vi "N-Double FFT Mesurament (N-Parametric) Test.vi"() -> ()   [LabVIEW 2014]
uses:
  <vilib>/Platform/TimedLoop/XDataNode/timing_clust.ctl
  <vilib>/Platform/TimedLoop/XDataNode/nitl_modes.ctl
  <vilib>/Platform/TimedLoop/XDataNode/wakeup.ctl
  <vilib>/rvi/Analysis/measure/FFT/simModelSupport/niFPGA FFT Streaming Sim Properties.ctl
  <vilib>/rvi/Analysis/measure/FFT/simModelSupport/niFPGA FFT Sim Stream Group Properties.ctl
  <vilib>/rvi/Analysis/measure/FFT/simModelSupport/niFPGA FFT Sim Types.ctl
  <vilib>/rvi/Analysis/measure/FFT/simModelSupport/niFpgaFFTSimArithmeticProperties.ctl
  <vilib>/rvi/Analysis/measure/FFT/simModelSupport/niFpgaFFTSimDfxp.ctl
  <vilib>/fxp/LVFixedPointQuantizationPolicyTypeDef.ctl
  <vilib>/rvi/Analysis/measure/FFT/XNode/niFpgaFFTButterflyDelays.ctl
  <vilib>/rvi/Emulation/niFpgaSctlEmulationGetInTimedLoop.vi
  <vilib>/rvi/Emulation/niFpgaEmulationReportErrorSimple.vi
  <vilib>/rvi/Emulation/niFpgaGetClockAttributes.vi
  <vilib>/rvi/Emulation/niFpgaCriticalErrorInLSC.vi
  <vilib>/rvi/Emulation/niFpgaEmulationIsFPGAContextNoSignature.vi
  <vilib>/rvi/DataTransferAndStorage/Container/Common/niFpgaContainerGetUniqueNameForEmu.vi
  <vilib>/rvi/Memory/Memory_Emulation/niFpgaMemoryEmulationCacheClearOnFirstRun.vi
  <vilib>/rvi/Memory/Memory_Emulation/nirvimemoryEmulationManagerCache_MakeExclusive.vi
  <vilib>/rvi/Memory/Memory_Emulation/niFpgaMemoryEmulationValidateCache.vi
  <vilib>/rvi/Memory/Memory_Emulation/nirvimemoryEmulationManagerCache_InsertValue.vi
  <vilib>/Utility/error.llb/Clear Errors.vi
  <vilib>/rvi/Memory/Memory_Emulation/nirvimemoryEmulationManagerCache_ReleaseExclusive.vi
  <vilib>/rvi/Memory/Memory_Emulation/nirvimemoryEmulationManagerCache_GetValue.vi
  <vilib>/rvi/Memory/Memory_Emulation/nirvimemoryEmulationManagerCache_SetValue.vi
  <vilib>/rvi/Emulation/niFpgaProcessEmulError.vi
  <vilib>/rvi/errors/niFpgaSetErrorForExecOnDevCompSimple.vi
  <vilib>/rvi/eio/common/nirviEmuReportErrorAndStop.vi
  <vilib>/rvi/FIFO/Fifo_Resource/nirvififoEmulationSetSize.vi
  <vilib>/rvi/FIFO/Fifo_Resource/nirviFifoEmulationQueueMgr.vi
  <instcachedir>/0/nirviFifoEmulationQueueMgr_E5CAEC123FF24DC58D834DCA3CDAA9B5.lvgen/nirviFifoEmulationQueueMgr_E5CAEC123FF24DC58D834DCA3CDAA9B5_010.vi
  <vilib>/rvi/FIFO/Fifo_Resource/nirvififoEmulationCreateLock.vi
  <vilib>/rvi/FIFO/Fifo_Resource/nirvififoEmulationObtainLock.vi
  <vilib>/rvi/FIFO/Fifo_Resource/nirvififoEmulationReleaseLock.vi
  <vilib>/rvi/occurrence/nirviWaitOnOccurrenceBase.vi
  <vilib>/rvi/errors/nirviReportUnexpectedCaseInternalError.vi
  <vilib>/rvi/errors/nirviReportUnexpectedCaseInternalError (U32).vi
  <vilib>/rvi/FIFO/Fifo_Resource/nirvififoEmulationDetermineInputValidOut.vi
  <vilib>/rvi/Memory/Memory_Emulation/nirvimemoryFastEmulation.vi
  <vilib>/rvi/Memory/Memory_Emulation/nirvimemoryEmulation.vi
  <vilib>/rvi/eio/common/nirviEmuTemplateMethod_errors.vi
  <vilib>/rvi/Analysis/measure/FFT/simModelSupport/niFpgaFFTSimModelStreamingCore.vi
  <vilib>/rvi/interface/RandomDataEmulation/niFpgaRandomDataHandleErrors.vi
  <vilib>/Platform/TimedLoop/XDataNode/XDataNode.xnode
  <vilib>/rvi/DataTransferAndStorage/Container/XNode/niFpgaContainer.xnode
  <vilib>/rvi/DataTransferAndStorage/Register/Emulation/niFpgaRegisterEmulation.vi
  <vilib>/rvi/FIFO/Fifo_Resource/nirvififoEmulationRead.vi
  <vilib>/rvi/FIFO/Fifo_Resource/nirvififoEmulationWrite.vi
  <vilib>/eio/EIOMethodNode/EIOMethodNode.xnode
  <vilib>/rvi/Analysis/measure/FFT/XNode/niFpgaFFT.xnode
  <vilib>/rvi/interface/RandomDataEmulation/nirviRandomDataFpgaReadWriteTemplate.vi
  <vilib>/Platform/TimedLoop/XDataNode/XDNodeRunTimeDep.lvlib
panel:
  in  "n":u32=1
  in  "Latency points":u32
  in  "snapshot":bool
  in  "lower limit 2":u32=682
  in  "lower limit 1":u32=57
  in  "upper limit 2":u32=1193
  in  "upper limit 1":u32=568
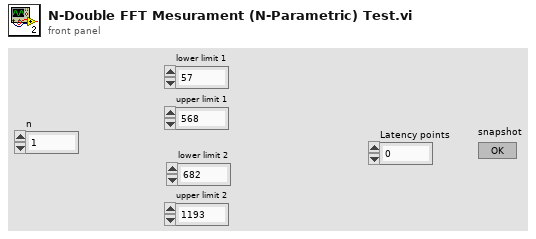
[diagram p1: front panel]
types:
  T1 = typedef "XDNodeRunTimeDep.lvlib/timing_clust.ctl" = cluster{"Expected End [f-1]":u64, "Actual End [f-1]":u64, "Finished Late? [f-1]":bool, "Expected End [i-1]":u64, "Actual End [i-1]":u64, "Finished Late? [i-1]":bool, "Expected Start [i]":u64, "Actual Start [i]":u64, "Expected Start [f]":u64, "Actual Start [f]":u64, "Source Name":string, "Structure Name":string, "Period":i64, "Deadline":i64, "Offset":i64, "Start":i64, "Priority":i32, "Timeout":i32, "Mode":T2, "Wakeup Reason":T3, "Error":errorcluster, "Source Type":string, "Secondary Source Type":string, "Global End Time":u64, "Global Start Time":u64, "Frame Duration":u64, "Iteration Duration":u64, "Assigned CPU":i32, "I/O Scan Engine Mode":u32}
  T2 = typedef "XDNodeRunTimeDep.lvlib/nitl_modes.ctl" = enum32{"No Change", "Process missed periods, maintain original phase", "Discard missed periods, maintain original phase", "Process missed periods, ignore original phase", "Discard missed periods, ignore original phase"}
  T3 = typedef "XDNodeRunTimeDep.lvlib/wakeup.ctl" = enum32{"Normal", "Aborted", "Asynchronous wakeup", "Timing source error", "Timed loop error", "Timeout"}
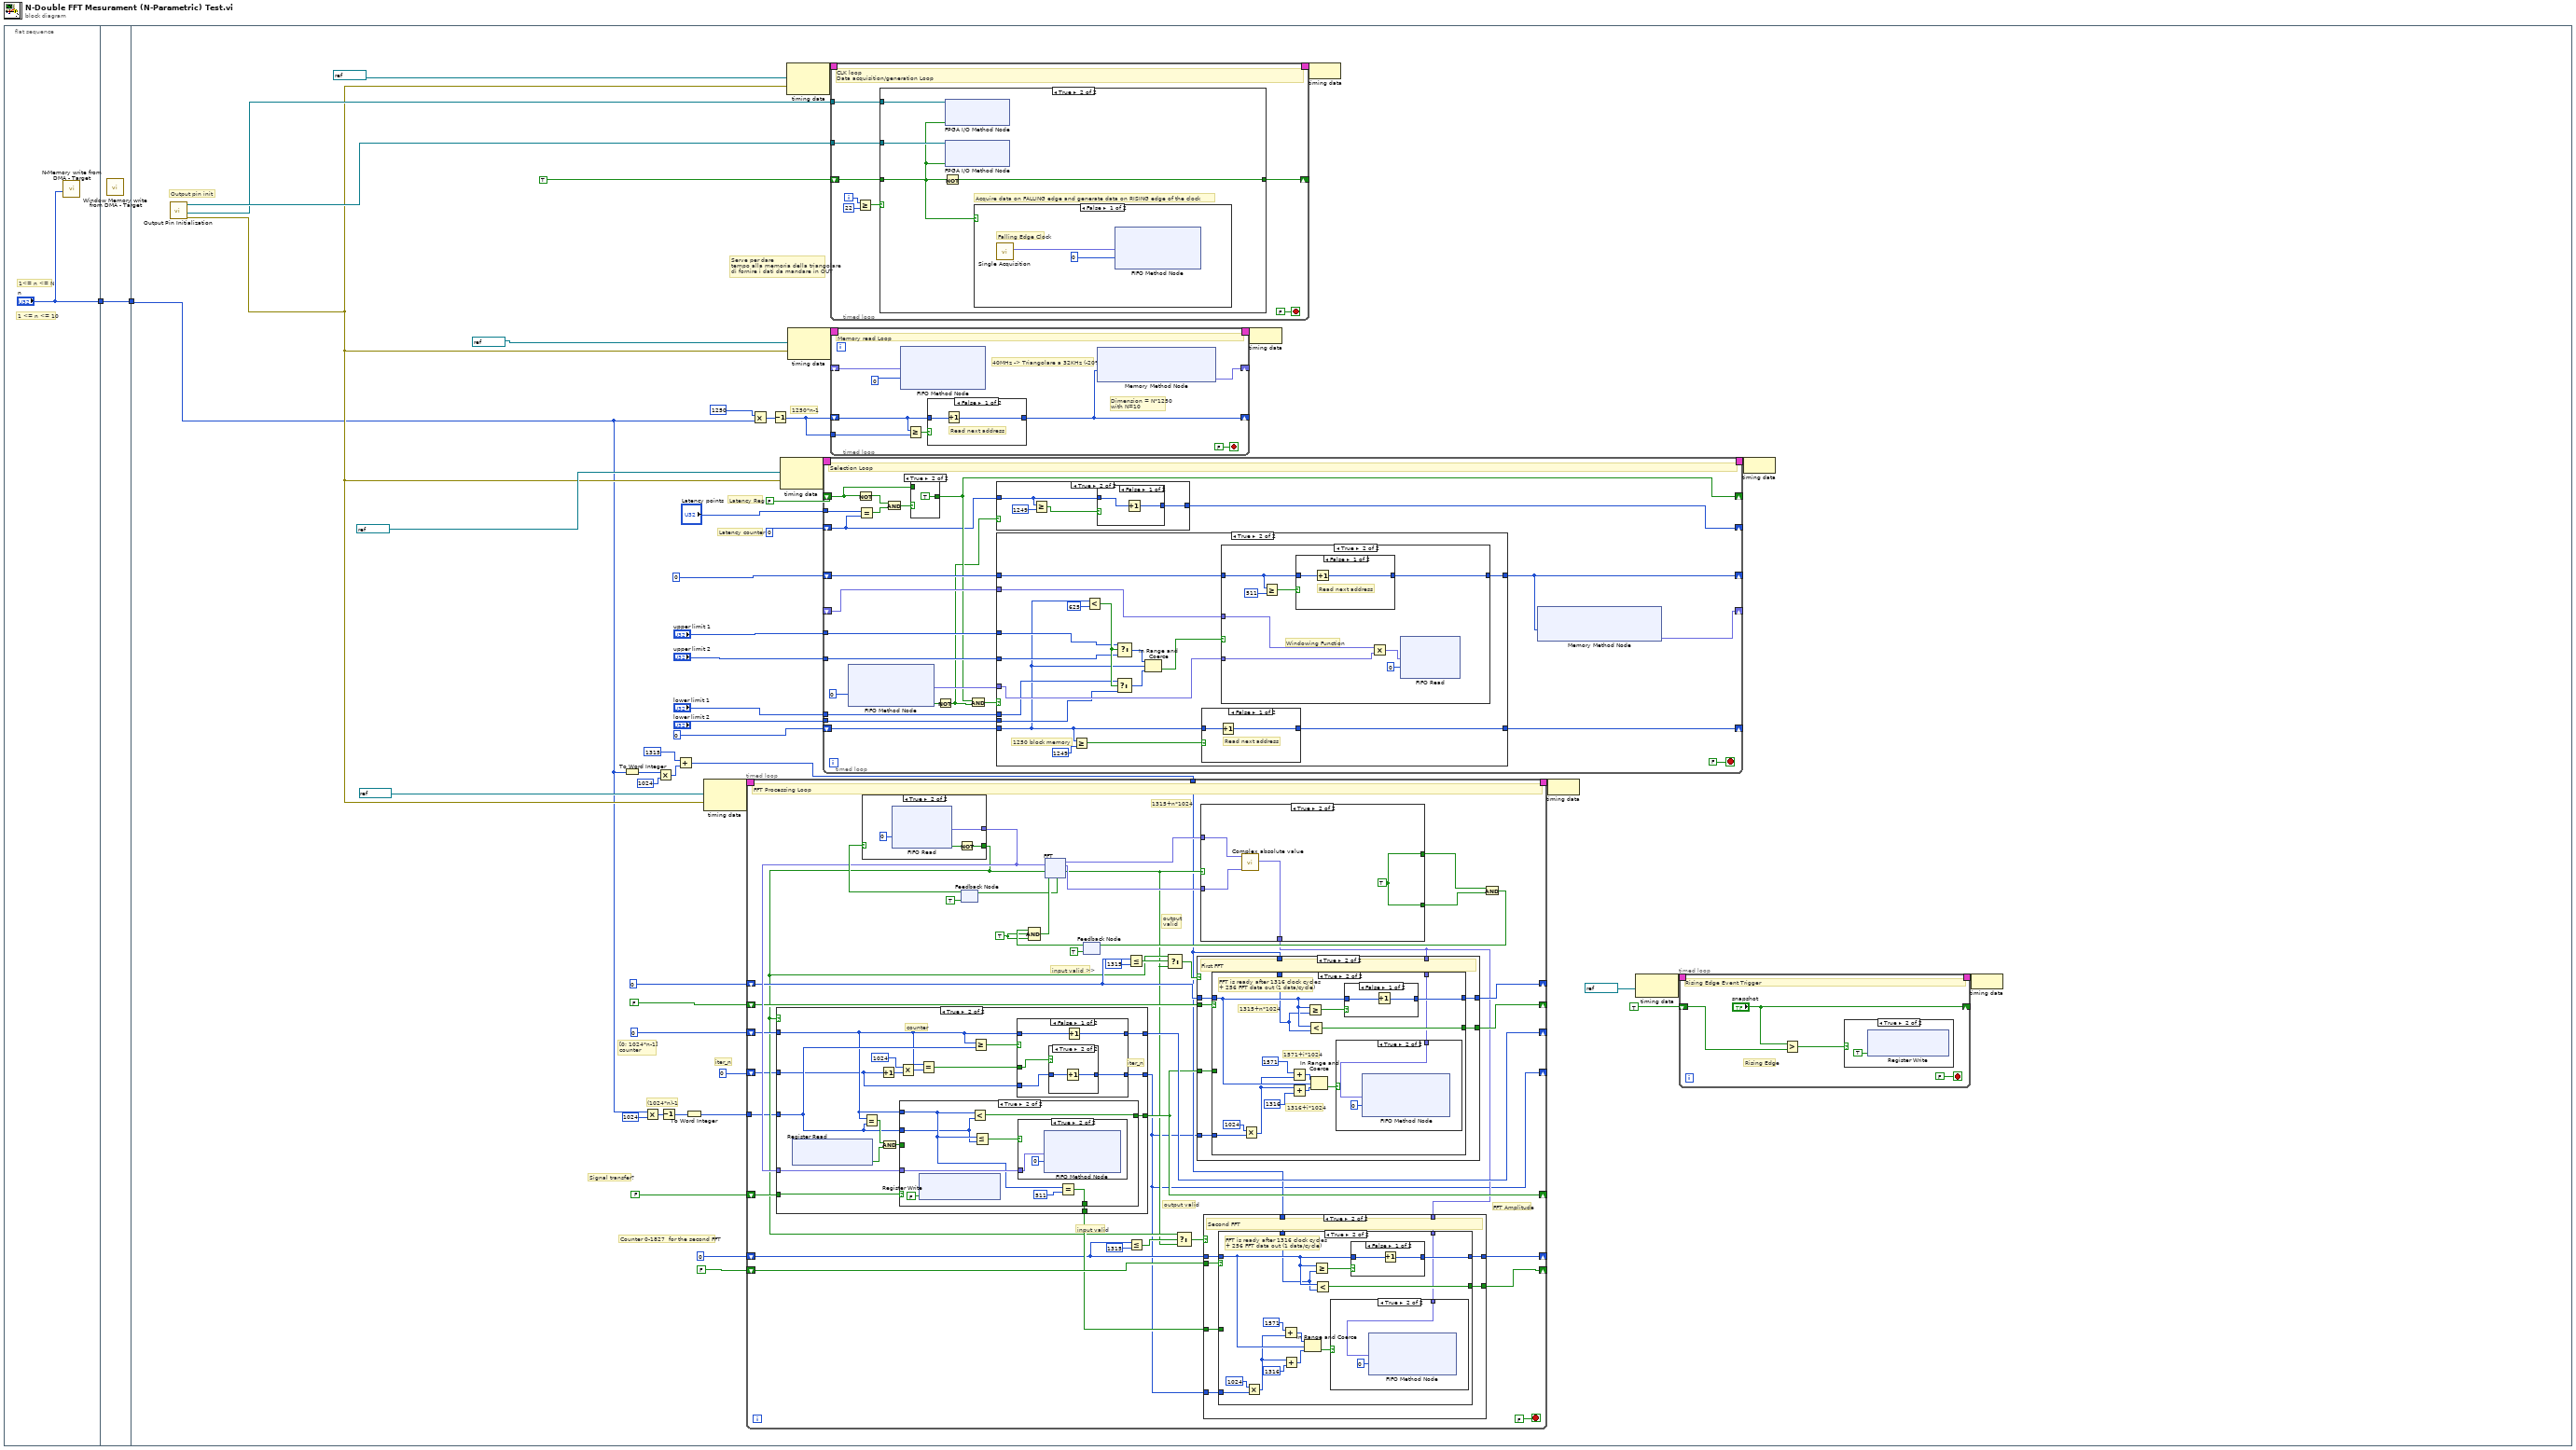
[diagram p0: block diagram]
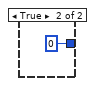
[diagram p4: hidden frame]
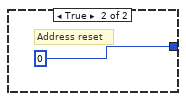
[diagram p8: hidden frame]
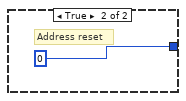
[diagram p9: hidden frame]
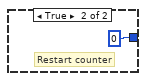
[diagram p13: hidden frame]
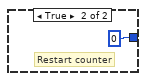
[diagram p17: hidden frame]
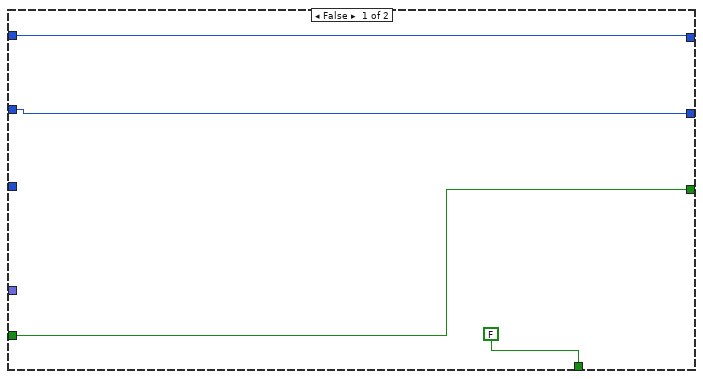
[diagram p18: hidden frame]
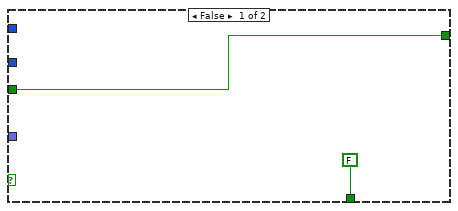
[diagram p19: hidden frame]
diagram:
  n1 = flat-sequence {
    tunnel: ["n"] -> w1
    tunnel: [w4] -> w2
    tunnel: w1 -> [w4]
    tunnel: w2 -> [w6]
    frame #0 {
      # "1 <= n <= 10"
      # "1<= n <= N"
      n2 = call "N-Memory write from DMA - Target.vi"("n"="n") -> ()  [unwired: 11 in]
    }
    frame #1 {
      n3 = call "Window Memory write from DMA - Target.vi"() -> ()  [unwired: 12 in]
    }
    frame #2 {
      # "iter_n"
      # "(1024*n)-1"
      # "1250*n-1"
      # "Serve per dare\ntempo alla memoria della triangolare\ndi fornire i dati da mandare in OUT"
      # "Latency counter"
      # "Latency Reg"
      # "Counter 0-1827  for the second FFT"
      # "[0; 1024*n-1]\ncounter"
      # "Signal transfer?"
      # "Output pin init"
      n4 = call "Output Pin Initialization.vi"() -> ("error out"=w37:errorcluster, "I/O Out Clock DAC (pin16)"=w41:refnum<k21>, "I/O Out Clock ADC (pin17)"=w42:refnum<k21>)  [unwired: 8 in]
      n5 = To Word Integer(number=w6) -> (16bit integer=w7:i16)
      n6 = Multiply(x=w6, y=u32 1024) -> (x*y=w14:u32)
      n7 = Multiply(x=w7, y=i16 1024) -> (x*y=w9:i16)
      n8 = Decrement(x=w14) -> (x-1=w13:u32)
      n9 = Add(x=i16 1315 ("y"), y=w9) -> (x+y=w5:i16)
      n10 = To Word Integer(number=w13) -> (16bit integer=w12:i16)
      n11 = node-c288(refnum<k21> "40MHz" ("Source Name"), w37) -> (w49:T1)
      n12 = timed-loop {
        timing: w49 -> [_]
        timing-out: [_] -> w48
        shift-right: [w163] -> _
        shift-left: FALSE -> [w166]
        shift-right: [w167] -> _
        shift-left: i16 0 -> [w164]
        shift-right: [w162] -> _
        shift-left: FALSE -> [w161]
        shift-right: [w160] -> _
        shift-left: i16 0 -> [w158]
        shift-right: [w155] -> _
        shift-left: i16 0 -> [w148]
        shift-right: [w152] -> _
        shift-left: FALSE -> [w153]
        tunnel: w12 -> [w143]
        shift-right: [w140] -> _
        shift-left: i16 0 -> [w142]
        tunnel: w5 -> [w141]
        stop <- FALSE stop-if-true
        w144 = TRUE
        # "1315+n*1024"
        # "output valid"
        # "input valid"
        # "FFT Amplitude"
        # "output\nvalid"
        # "input valid >>"
        # "FFT Processing Loop"
        n13 = feedback #1(TRUE ("ready for input")) -> (w179:bool)
        n14 = case shown="True" w179 {
          tunnel: [FALSE w320] -> w147
          tunnel: [fxp<+/-,12,12> 0.0 ("Element") w317] -> w165
          frame False {
            # "RMS is not ready for new input"
          }
          frame True {
            n15 = xnode ("FIFO Read")("Timeout"=0) -> ("Element"=w317:fxp<+/-,12,12>, "Timed Out?"=w319:bool)  [unwired: 1 in, 1 out]
            n16 = Not(x=w319) -> (.not. x?=w320:bool)
          }
        }
        n17 = case shown="True" w147 {
          tunnel: w164 -> [w245 w249]
          tunnel: [w245 w261] -> w167
          tunnel: w166 -> [w244 w257]
          tunnel: [w244 w258] -> w163
          tunnel: w165 -> [_ w256]
          tunnel: [FALSE w254] -> w151
          tunnel: w143 -> [_ w253]
          tunnel: w142 -> [w242 w247]
          tunnel: [w242 w246] -> w140
          frame False {
          }
          frame True {
            # "iter_n"
            # "counter"
            n18 = xnode ("Register Read")() -> ("Data"=w255:bool)  [unwired: 1 in, 1 out]
            n19 = Equal?(x=w249, y=w253) -> (x = y?=w260:bool)
            n20 = Increment(x=w247) -> (x+1=w252:i16)
            n21 = And(x=w260, y=w255) -> (x .and. y?=w259:bool)
            n22 = Multiply(x=i16 1024, y=w252) -> (x*y=w250:i16)
            n23 = case shown="True" w257 {
              tunnel: w259 -> [w264 _]
              tunnel: w249 -> [_ w266]
              tunnel: [w264 w272] -> w258
              tunnel: w256 -> [_ w267]
              tunnel: [FALSE w268] -> w254
              tunnel: w253 -> [_ w265]
              frame False {
              }
              frame True {
                n24 = xnode ("Register Write")("Data"=FALSE) -> ()  [unwired: 1 in, 1 out]
                n25 = Less?(x=w266, y=w265) -> (x < y?=w272:bool)
                n26 = Less Or Equal?(x=w266, y=w265) -> (x <= y?=w271:bool)
                n27 = case shown="True" w271 {
                  tunnel: w267 -> [_ w273]
                  frame False {
                  }
                  frame True {
                    n28 = xnode ("FIFO Method Node")("Element"=w273, "Timeout"=0) -> ()  [unwired: 1 in, 2 out]
                  }
                }
                n29 = Equal?(x=w266, y=i16 511) -> (x = y?=w268:bool)
              }
            }
            n30 = Equal?(x=w249, y=w250) -> (x = y?=w248:bool)
            n31 = Greater Or Equal?(x=w249, y=w253) -> (x >= y?=w262:bool)
            n32 = case shown="False" w262 {
              tunnel: w249 -> [w279 _]
              tunnel: [w278 w283] -> w261
              tunnel: w248 -> [w276 _]
              tunnel: w247 -> [w277 _]
              tunnel: [w275 w283] -> w246
              frame False {
                n33 = case shown="True" w276 {
                  tunnel: w277 -> [w280 w282]
                  tunnel: [w280 w281] -> w275
                  frame False {
                  }
                  frame True {
                    n34 = Increment(x=w282) -> (x+1=w281:i16)
                  }
                }
                n35 = Increment(x=w279) -> (x+1=w278:i16)
              }
              frame True {
                w283 = i16 0
                # "Restart counter"
              }
            }
          }
        }
        n36 = feedback #2(TRUE) -> (w175:bool)
        n37 = Compound Arithmetic op=AND(w175, w144, w144) -> (w174:bool)
        n38 = xnode "FFT"("real data in"=w165, "input valid"=w147, "ready for output"=w174) -> ("ready for input"=w173:bool, "real data out"=w172:fxp<+/-,22,22>, "imaginary data out"=w171:fxp<+/-,22,22>, "output valid"=w145:bool)  [unwired: 2 in, 1 out]
        n39 = feedback-in #1(w173) -> ()
        n40 = Less Or Equal?(x=w158, y=i16 1315) -> (x <= y?=w159:bool)
        n41 = Less Or Equal?(x=w148, y=i16 1315) -> (x <= y?=w149:bool)
        n42 = Select(t=w147, s=w159, f=w145) -> (s? t:f=w156:bool)
        n43 = Select(t=w147, s=w149, f=w145) -> (s? t:f=w146:bool)
        n44 = case shown="True" w145 {
          tunnel: w172 -> [_ w314]
          tunnel: w171 -> [_ w313]
          tunnel: [w310 w311] -> w170
          tunnel: [w310 w311] -> w169
          tunnel: [_ w312] -> w154
          frame False {
            w310 = TRUE
          }
          frame True {
            w311 = TRUE
            n45 = call "Complex absolute value.vi"("Im"=w313, "Re"=w314) -> ("Square Absolute Value"=w312:fxp<+,44,44>)  [unwired: 9 in]
          }
        }
        n46 = case shown="True" w156 {
          tunnel: w163 -> [_ w220]
          tunnel: [w211 w219] -> w162
          tunnel: w161 -> [w211 w218]
          tunnel: w158 -> [w212 w217]
          tunnel: [w212 w216] -> w160
          tunnel: w154 -> [_ w215]
          tunnel: w141 -> [_ w214]
          tunnel: w140 -> [_ w213]
          frame False {
          }
          frame True {
            # "First FFT"
            n47 = case shown="True" w218 {
              tunnel: w220 -> [w222 _]
              tunnel: [w222 w236] -> w219
              tunnel: w217 -> [w221 w231]
              tunnel: [w221 w234] -> w216
              tunnel: w215 -> [_ w232]
              tunnel: w214 -> [_ w230]
              tunnel: w213 -> [_ w224]
              frame False {
              }
              frame True {
                # "1571+i*1024"
                # "1316+i*1024"
                # "1315+n*1024"
                # "FFT is ready after 1316 clock cycles\n+ 256 FFT data out (1 data/cycle)"
                n48 = Multiply(x=i16 1024 ("upper limit"), y=w224) -> (x*y=w223:i16)
                n49 = Add(x=i16 1571 ("upper limit"), y=w223) -> (x+y=w227:i16)
                n50 = Add(x=w223, y=i16 1316) -> (x+y=w229:i16)
                n51 = Greater Or Equal?(x=w231, y=w230) -> (x >= y?=w235:bool)
                n52 = Less?(x=w231, y=w230) -> (x < y?=w236:bool)
                n53 = In Range and Coerce(upper limit=w227, x=w231, lower limit=w229) -> (In Range?=w233:bool)  [unwired: 1 out]
                n54 = case shown="True" w233 {
                  tunnel: w232 -> [_ w238]
                  frame False {
                  }
                  frame True {
                    n55 = xnode ("FIFO Method Node")("Element"=w238, "Timeout"=0) -> ()  [unwired: 1 in, 2 out]
                  }
                }
                n56 = case shown="False" w235 {
                  tunnel: w231 -> [w240 _]
                  tunnel: [w239 i16 0] -> w234
                  frame False {
                    n57 = Increment(x=w240) -> (x+1=w239:i16)
                  }
                  frame True {
                    # "Restart counter"
                  }
                }
              }
            }
          }
        }
        n58 = case shown="True" w146 {
          tunnel: w151 -> [_ w189]
          tunnel: [w180 w188] -> w152
          tunnel: w153 -> [w180 w187]
          tunnel: w148 -> [w181 w186]
          tunnel: [w181 w185] -> w155
          tunnel: w154 -> [_ w184]
          tunnel: w141 -> [_ w183]
          tunnel: w140 -> [_ w182]
          frame False {
          }
          frame True {
            # "Second FFT"
            n59 = case shown="True" w187 {
              tunnel: w189 -> [w191 _]
              tunnel: [w191 w205] -> w188
              tunnel: w186 -> [w190 w202]
              tunnel: [w190 w203] -> w185
              tunnel: w184 -> [_ w200]
              tunnel: w183 -> [_ w199]
              tunnel: w182 -> [_ w197]
              frame False {
              }
              frame True {
                # "FFT is ready after 1316 clock cycles\n+ 256 FFT data out (1 data/cycle)"
                n60 = Multiply(x=i16 1024 ("upper limit"), y=w197) -> (x*y=w192:i16)
                n61 = Add(x=i16 1571 ("upper limit"), y=w192) -> (x+y=w193:i16)
                n62 = Add(x=w192, y=i16 1316) -> (x+y=w195:i16)
                n63 = In Range and Coerce(upper limit=w193, x=w202, lower limit=w195) -> (In Range?=w201:bool)  [unwired: 1 out]
                n64 = Greater Or Equal?(x=w202, y=w199) -> (x >= y?=w204:bool)
                n65 = Less?(x=w202, y=w199) -> (x < y?=w205:bool)
                n66 = case shown="True" w201 {
                  tunnel: w200 -> [_ w207]
                  frame False {
                  }
                  frame True {
                    n67 = xnode ("FIFO Method Node")("Element"=w207, "Timeout"=0) -> ()  [unwired: 1 in, 2 out]
                  }
                }
                n68 = case shown="False" w204 {
                  tunnel: w202 -> [w209 _]
                  tunnel: [w208 i16 0] -> w203
                  frame False {
                    n69 = Increment(x=w209) -> (x+1=w208:i16)
                  }
                  frame True {
                    # "Restart counter"
                  }
                }
              }
            }
          }
        }
        n70 = Compound Arithmetic op=AND(w170, w169) -> (w168:bool)
        n71 = feedback-in #2(w168) -> ()
      }
      n72 = Multiply(x=u32 1250, y=w6) -> (x*y=w17:u32)
      n73 = Decrement(x=w17) -> (x-1=w16:u32)
      n74 = node-c288(refnum<k21> "40MHz" ("Source Name"), w37) -> (w47:T1)
      n75 = node-c288(refnum<k21> "80MHz" ("Source Name"), w37) -> (w53:T1)
      n76 = node-c288(refnum<k21> "40MHz" ("Source Name"), w37) -> (w51:T1)
      n77 = timed-loop {
        timing: w47 -> [_]
        timing-out: [_] -> w46
        shift-right: [w87] -> _
        shift-left: u32 0 -> [w74]
        tunnel: "upper limit 1" -> [w83]
        tunnel: "upper limit 2" -> [w82]
        tunnel: "lower limit 1" -> [w81]
        tunnel: "lower limit 2" -> [w80]
        shift-right: [w76] -> _
        shift-left: u32 0 -> [w79]
        shift-right: [w77] -> _
        shift-left: _ -> [w78]
        shift-right: [w68] -> _
        shift-left: FALSE -> [w69]
        tunnel: "Latency points" -> [w73]
        shift-right: [w66] -> _
        shift-left: u32 0 -> [w65]
        stop <- FALSE stop-if-true
        # "Selection Loop"
        n78 = xnode ("FIFO Method Node")("Timeout"=0) -> ("Element"=w85:fxp<+/-,12,12>, "Timed Out?"=w86:bool)  [unwired: 1 in, 1 out]
        n79 = Not(x=w69) -> (.not. x?=w72:bool)
        n80 = Equal?(x=w73, y=w65) -> (x = y?=w71:bool)
        n81 = And(x=w72, y=w71) -> (x .and. y?=w70:bool)
        n82 = case shown="True" w70 {
          tunnel: [w97 TRUE] -> w68
          tunnel: w69 -> [w97 _]
          frame False {
          }
          frame True {
          }
        }
        n83 = Not(x=w86) -> (.not. x?=w67:bool)
        n84 = And(x=w68, y=w67) -> (x .and. y?=w75:bool)
        n85 = case shown="True" w67 {
          tunnel: w65 -> [w89 w92]
          tunnel: [w89 w90] -> w66
          frame False {
          }
          frame True {
            n86 = Greater Or Equal?(x=w92, y=u32 1249) -> (x >= y?=w91:bool)
            n87 = case shown="False" w91 {
              tunnel: w92 -> [w95 _]
              tunnel: [w94 u32 0] -> w90
              frame False {
                n88 = Increment(x=w95) -> (x+1=w94:u32)
              }
              frame True {
              }
            }
          }
        }
        n89 = case shown="True" w75 {
          tunnel: [w100 w115] -> w87
          tunnel: w74 -> [w100 w102]
          tunnel: w85 -> [_ w110]
          tunnel: w83 -> [_ w109]
          tunnel: w82 -> [_ w108]
          tunnel: w81 -> [_ w107]
          tunnel: w80 -> [_ w106]
          tunnel: w79 -> [w99 w103]
          tunnel: [w99 w105] -> w76
          tunnel: w78 -> [_ w104]
          frame False {
          }
          frame True {
            # "1250 block memory"
            n90 = Greater Or Equal?(x=w102, y=u32 1249) -> (x >= y?=w116:bool)
            n91 = Less?(x=w102, y=u32 625) -> (x < y?=w111:bool)
            n92 = Select(t=w107, s=w111, f=w106) -> (s? t:f=w113:u32)
            n93 = Select(t=w109, s=w111, f=w108) -> (s? t:f=w114:u32)
            n94 = In Range and Coerce(upper limit=w114, x=w102, lower limit=w113) -> (In Range?=w101:bool)  [unwired: 1 out]
            n95 = case shown="False" w116 {
              tunnel: w102 -> [w131 _]
              tunnel: [w130 u32 0] -> w115
              frame False {
                # "Read next address"
                n96 = Increment(x=w131) -> (x+1=w130:u32)
              }
              frame True {
                # "Address reset"
              }
            }
            n97 = case shown="True" w101 {
              tunnel: w110 -> [_ w119]
              tunnel: w103 -> [w118 w124]
              tunnel: [w118 w126] -> w105
              tunnel: w104 -> [_ w122]
              frame False {
              }
              frame True {
                # "Windowing Function"
                n98 = Greater Or Equal?(x=w124, y=u32 511) -> (x >= y?=w125:bool)
                n99 = case shown="False" w125 {
                  tunnel: w124 -> [w128 _]
                  tunnel: [w127 u32 0] -> w126
                  frame False {
                    # "Read next address"
                    n100 = Increment(x=w128) -> (x+1=w127:u32)
                  }
                  frame True {
                    # "Address reset"
                  }
                }
                n101 = Multiply(x=w122, y=w119) -> (x*y=w120:fxp<+/-,12,12>)
                n102 = xnode ("FIFO Read")("Element"=w120, "Timeout"=0) -> ()  [unwired: 1 in, 2 out]
              }
            }
          }
        }
        n103 = xnode ("Memory Method Node")("Address"=w76) -> ("Data"=w77:fxp<+,8,1>)  [unwired: 1 in, 1 out]
      }
      n104 = timed-loop {
        timing: w53 -> [_]
        timing-out: [_] -> w52
        shift-right: [w351] -> _
        shift-left: TRUE -> [w349]
        tunnel: w41 -> [w353]
        tunnel: w42 -> [w350]
        i -> [w347]
        stop <- FALSE stop-if-true
        # "CLK loop\nData acquisition/generation Loop"
        n105 = Greater Or Equal?(x=w347, y=22) -> (x >= y?=w346:bool)
        n106 = case shown="True" w346 {
          tunnel: w353 -> [_ w358]
          tunnel: [w354 w357] -> w351
          tunnel: w350 -> [_ w356]
          tunnel: w349 -> [w354 w355]
          frame False {
          }
          frame True {
            # "Acquire data on FALLING edge and generate data on RISING edge of the clock"
            n107 = Not(x=w355) -> (.not. x?=w357:bool)
            n108 = xnode "FPGA I/O Method Node"("FPGA I/O In"=w358, "Data"=w355) -> ()  [unwired: 1 out]
            n109 = xnode "FPGA I/O Method Node"("FPGA I/O In"=w356, "Data"=w355) -> ()  [unwired: 1 out]
            n110 = case shown="False" w355 {
              frame False {
                # "Falling Edge Clock"
                n111 = call "Single Acquisition.vi"() -> ("Out"=w360:fxp<+/-,12,12>)  [unwired: 10 in, 1 out]
                n112 = xnode ("FIFO Method Node")("Element"=w360, "Timeout"=0) -> ()  [unwired: 1 in, 2 out]
              }
              frame True {
                # "Rising Edge Clock"
                n113 = xnode ("FIFO Method Node")("Timeout"=0) -> ("Element"=w361:fxp<+/-,12,12>, "Timed Out?"=w362:bool)  [unwired: 1 in, 1 out]
                n114 = case shown="False" w362 {
                  tunnel: w361 -> [w366 _]
                  frame False {
                    # "Data Generation"
                    n115 = Add(x=w366, y=fxp<+,12,12> 2048.0) -> (x+y=w364:fxp<+/-,14,14>)
                    n116 = call "Single Point Wave generation.vi"("Data To Write"=w364) -> ()  [unwired: 10 in, 1 out]
                  }
                  frame True {
                    # "FPGA memory slow"
                  }
                }
              }
            }
          }
        }
      }
      n117 = timed-loop {
        timing: w51 -> [_]
        timing-out: [_] -> w50
        shift-right: [w329] -> _
        shift-left: w16 -> [w333]
        shift-right: [w331] -> _
        shift-left: _ -> [w330]
        tunnel: w16 -> [w328]
        stop <- FALSE stop-if-true
        # "Dimension = N*1250\nwith N=10"
        # "40MHz -> Triangolare a 32KHz (-20%)"
        # "Memory read Loop"
        n118 = xnode ("FIFO Method Node")("Element"=w330, "Timeout"=0) -> ()  [unwired: 1 in, 2 out]
        n119 = Greater Or Equal?(x=w333, y=w328) -> (x >= y?=w335:bool)
        n120 = case shown="False" w335 {
          tunnel: w333 -> [w337 _]
          tunnel: [w336 u32 0] -> w329
          frame False {
            # "Read next address"
            n121 = Increment(x=w337) -> (x+1=w336:u32)
          }
          frame True {
            # "Address reset"
          }
        }
        n122 = xnode ("Memory Method Node")("Address"=w329) -> ("Data"=w331:fxp<+/-,12,12>)  [unwired: 1 in, 1 out]
      }
      n123 = node-c288(w50) -> ()
      n124 = node-c288(w52) -> ()
      n125 = node-c288(w48) -> ()
      n126 = node-c288(refnum<k21> "40MHz" ("Source Name")) -> (w27:T1)
      n127 = timed-loop {
        timing: w27 -> [_]
        timing-out: [_] -> w26
        shift-right: ["snapshot"] -> _
        shift-left: TRUE ("snapshot") -> [w56]
        stop <- FALSE stop-if-true
        # "Rising Edge"
        # "Rising Edge Event Trigger"
        n128 = Greater?(x="snapshot", y=w56) -> (0:w54:bool)
        n129 = case shown="True" w54 {
          frame False {
          }
          frame True {
            n130 = xnode ("Register Write")("Data"=TRUE) -> ()  [unwired: 1 in, 1 out]
          }
        }
      }
      n131 = node-c288(w46) -> ()
      n132 = node-c288(w26) -> ()
    }
  }
